vi "link -- generate comb.vi"(5 "maxY":dbl=1.0, 7 "minY":dbl, 8 "freq array":dbl[](array[numeric])) -> (0 "plot list":cluster{dbl[], dbl[]}[](array[cluster]), 1 "annotation list":T1(array[cluster]))   [LabVIEW 2014]
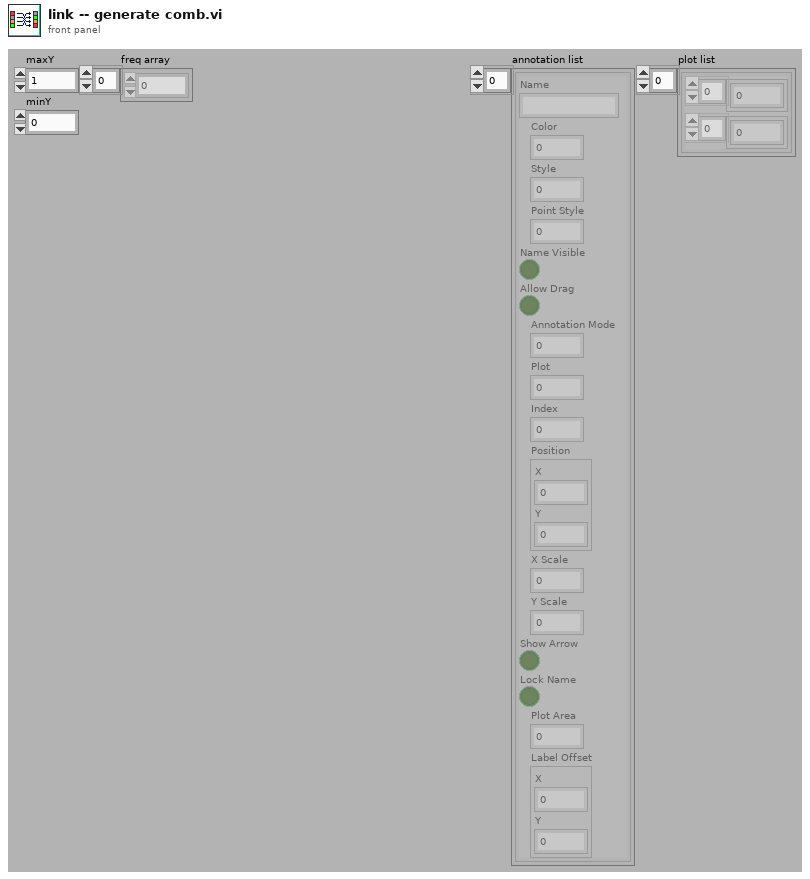
[diagram p1: front panel]
types:
  T1 = cluster{"Name":string, "Color":u32, "Style":u8, "Point Style":u8, "Name Visible":bool, "Allow Drag":bool, "Annotation Mode":u32, "Plot":i32, "Index":i32, "Position":cluster{"X":dbl, "Y":dbl}, "X Scale":u32, "Y Scale":u32, "Show Arrow":bool, "Lock Name":bool, "Plot Area":i32, "Label Offset":cluster{"X":dbl, "Y":dbl}}[]
  T2 = cluster{"Name":string, "Color":u32, "Style":u8, "Point Style":u8, "Name Visible":bool, "Allow Drag":bool, "Annotation Mode":u32, "Plot":i32, "Index":i32, "Position":cluster{"X":dbl, "Y":dbl}, "X Scale":u32, "Y Scale":u32, "Show Arrow":bool, "Lock Name":bool, "Plot Area":i32, "Label Offset":cluster{"X":dbl, "Y":dbl}}
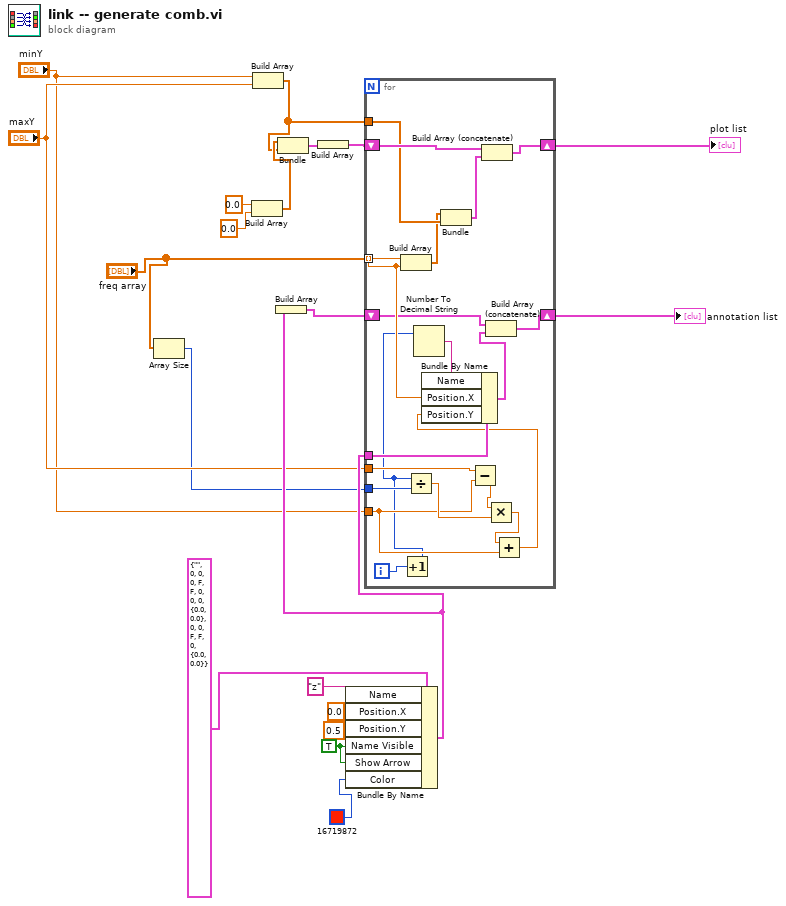
[diagram p0: block diagram]
diagram:
  w10 = TRUE ("Name Visible")
  n1 = Array Size(array="freq array") -> (size(s)=w2:i32)
  n2 = Build Array(0.0 ("element"), 0.0 ("element")) -> (w18:dbl[])
  n3 = Build Array("minY", "maxY") -> (w17:dbl[])
  n4 = Bundle(w18, w17) -> (w16:cluster{dbl[], dbl[]})  [unwired: 1 in]
  n5 = Build Array(w16) -> (w15:cluster{dbl[], dbl[]}[])
  n6 = Bundle By Name(cluster=T2 {"Name"="", "Color"=0, "Style"=0, "Point Style"=0, "Name Visible"=FALSE, "Allow Drag"=FALSE, "Annotation Mode"=0, "Plot"=0, "Index"=0, "Position"={"X"=0.0, "Y"=0.0}, "X Scale"=0, "Y Scale"=0, "Show Arrow"=FALSE, "Lock Name"=FALSE, "Plot Area"=0, "Label Offset"={"X"=0.0, "Y"=0.0}} ("element 2"), "Name"="z", "Position.X"=0.0, "Position.Y"=0.5, "Name Visible"=w10, "Show Arrow"=w10, "Color"=u32 16719872) -> (w6:T2)
  n7 = Build Array(w6) -> (w7:T1)
  n8 = for {
    shift-right: [w39] -> w1
    shift-left: w15 -> [w40]
    tunnel: w17 -> [w37]
    tunnel: "freq array" -> [w32] mode=indexing
    shift-right: [w35] -> w8
    shift-left: w7 -> [w30]
    tunnel: w6 -> [w34]
    tunnel: w2 -> [w29]
    tunnel: "maxY" -> [w28]
    tunnel: "minY" -> [w24]
    i -> [w22]
    n9 = Build Array(w32, w32) -> (w36:dbl[])
    n10 = Increment(x=w22) -> (x+1=w21:i32)
    n11 = Divide(x=w21, y=w29) -> (x/y=w26:dbl)
    n12 = Number To Decimal String(number=w21) -> (decimal integer string=w33:string)  [unwired: 1 in]
    n13 = Bundle(w36, w37) -> (w38:cluster{dbl[], dbl[]})  [unwired: 1 in]
    n14 = Subtract(x=w28, y=w24) -> (x-y=w27:dbl)
    n15 = Build Array (concatenate)(w40, w38) -> (w39:cluster{dbl[], dbl[]}[])
    n16 = Multiply(x=w27, y=w26) -> (x*y=w25:dbl)
    n17 = Add(x=w25, y=w24) -> (x+y=w23:dbl)
    n18 = Bundle By Name(cluster=w34, "Name"=w33, "Position.X"=w32, "Position.Y"=w23) -> (w31:T2)
    n19 = Build Array (concatenate)(w30, w31) -> (w35:T1)
  }
  "annotation list" <- w8
  "plot list" <- w1
